vi "get_voxel_trajectory.vi"(8 "error in (no error)":errorcluster, 11 "ScanHeadDL090202 in":refnum<class "ScanHeadDL090202.lvclass">) -> (0 "error out":errorcluster, 2 "trajectory":refnum<class "TrajectoryDL091126GenericVoxel.lvclass">, 3 "ScanHeadDL090202 out":refnum<class "ScanHeadDL090202.lvclass">)   [LabVIEW 2010, in "ScanHeadDL090202.lvclass"]
uses:
  ScanHeadDL090202.lvclass
  Trajectory/TrajectoryDL091126GenericVoxel/TrajectoryDL091126GenericVoxel/TrajectoryDL091126GenericVoxel.lvclass
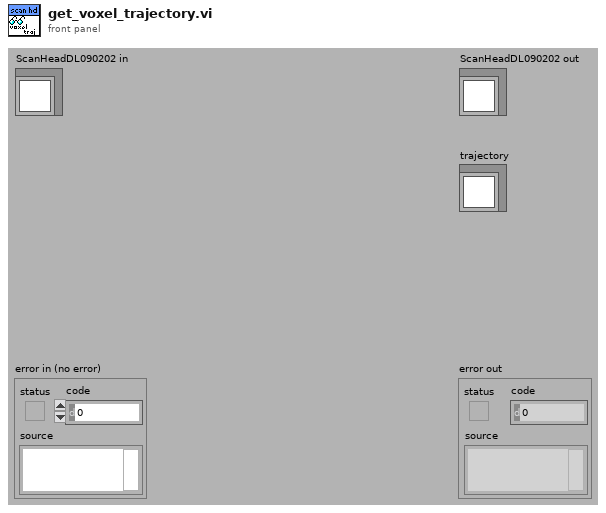
[diagram p1: front panel]
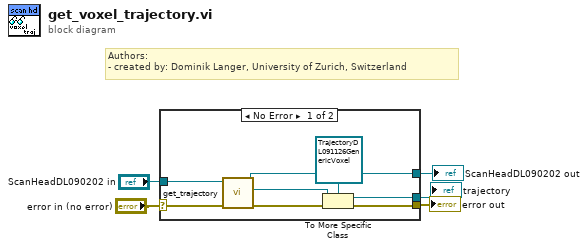
[diagram p0: block diagram]
diagram:
  # "Authors: \n- created by: Dominik Langer, University of Zurich, Switzerland"
  n1 = case shown="No Error" "error in (no error)" {
    selector: "error in (no error)" -> [w10 w15]
    tunnel: [w11 w15] -> w4
    tunnel: [w7 w14] -> w2
    tunnel: "ScanHeadDL090202 in" -> [w8 w14]
    tunnel: [w6 _] -> w1
    frame No Error {
      n2 = call-dynamic "get_trajectory.vi"("error in (no error)"=w10, "GenericScanHead.lvclass in"=w8) -> ("error out"=w9:errorcluster, "trajectory"=w12:refnum<class "GenericTrajectory.lvclass">, "GenericScanHead.lvclass out"=w7:refnum<class "ScanHeadDL090202.lvclass">)  [unwired: 7 in]
      n3 = To More Specific Class(target class=refnum<class "TrajectoryDL091126GenericVoxel.lvclass"> refnum ("TrajectoryDL091126GenericVoxel.lvclass"), reference=w12, error in=w9) -> (specific class reference=w6:refnum<class "TrajectoryDL091126GenericVoxel.lvclass">, error out=w11:errorcluster)
    }
    frame Error {
    }
  }
  "error out" <- w4
  "ScanHeadDL090202 out" <- w2
  "trajectory" <- w1
